vi "Sine_Trajectory_phase.vi"(6 "Phase(degrees)":dbl format="%0.2f", 7 "Amplitude":dbl, 8 "Offset":dbl, 9 "Frequency (Hz)":dbl, 10 "Duration (s)":dbl, 11 "Period (s)":dbl) -> (3 "Profile":cluster{"time (s)":dbl, "setpoint":dbl}[](array[cluster]) {"setpoint" format="%.2f"; "time (s)" format="%.3f"})   [LabVIEW 2015]
uses:
  <vilib>/Analysis/NI_AALBase.lvlib
panel:
  out "XY Graph":cluster{dbl, dbl}[](graph)
  # "Here needs to be 0.001 or so"
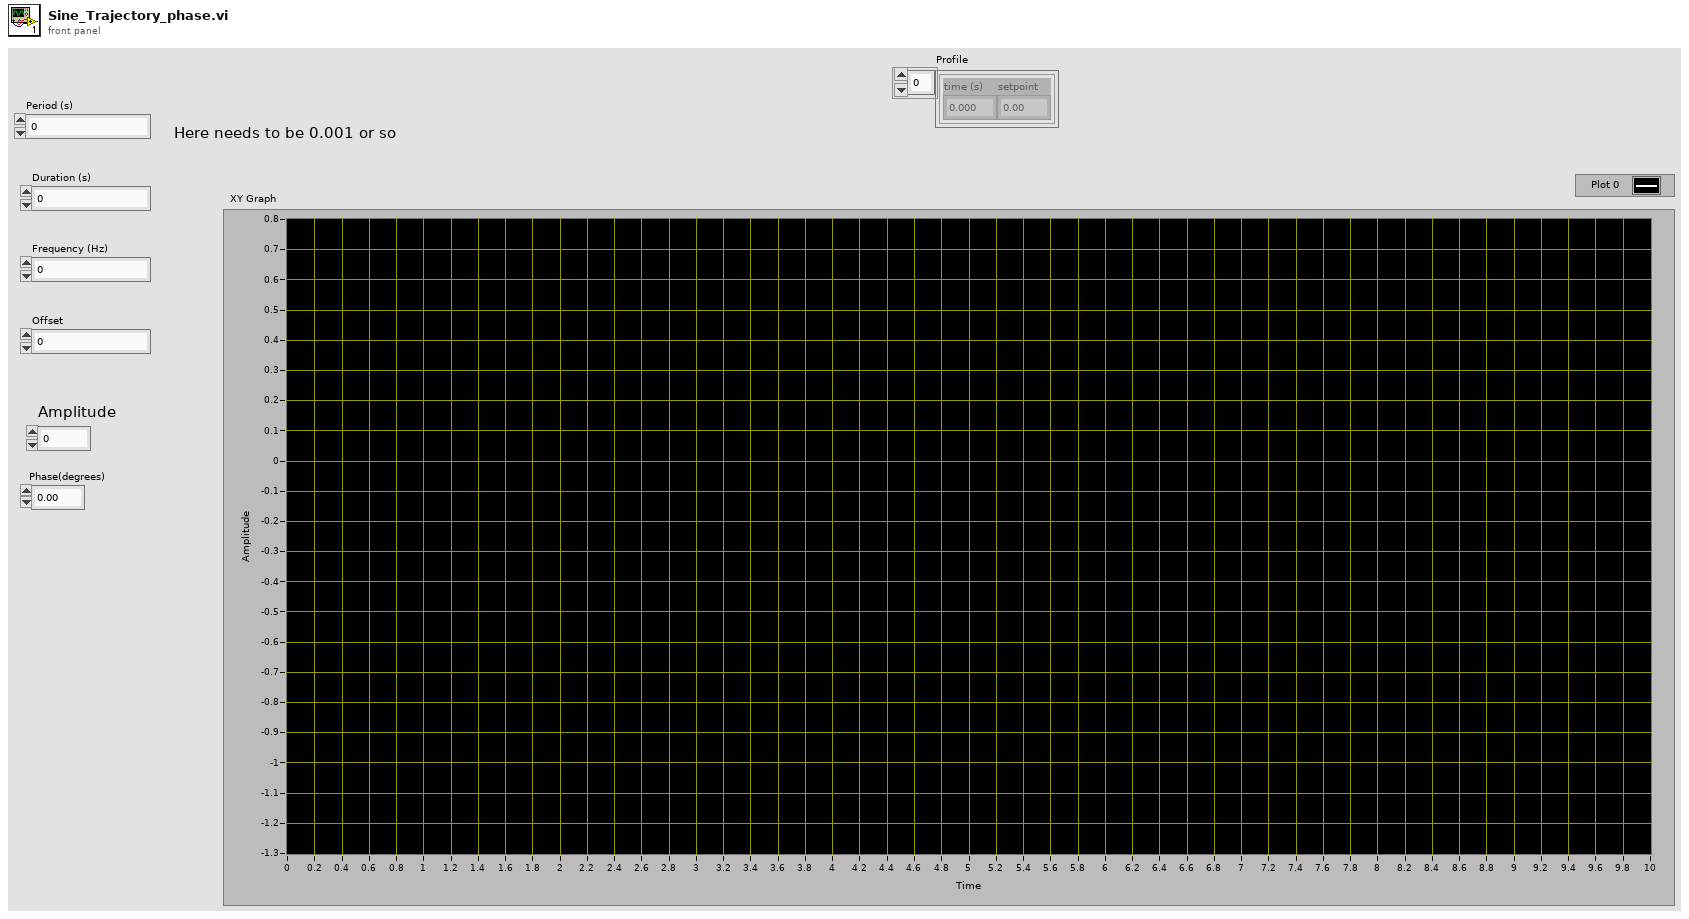
[diagram p1: front panel]
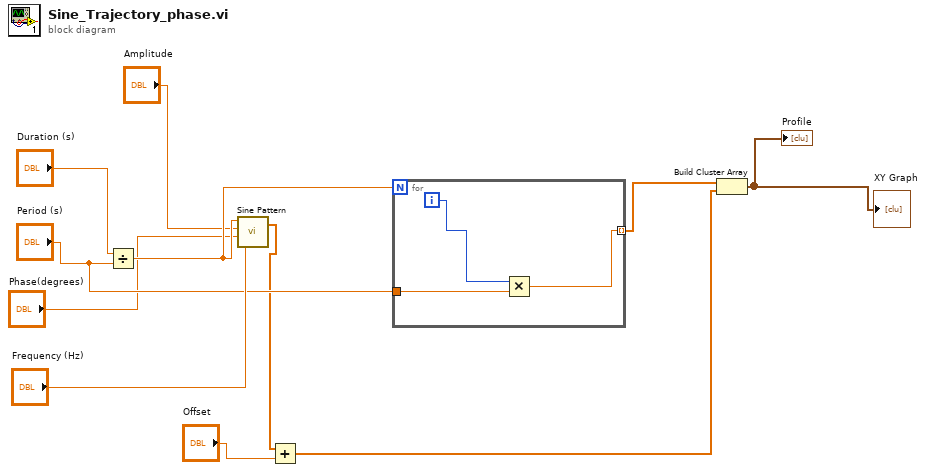
[diagram p0: block diagram]
diagram:
  n1 = Divide(x="Duration (s)", y="Period (s)") -> (x/y=w9:dbl)
  n2 = call <vilib>:"Sine Pattern.vi"("cycles"="Frequency (Hz)", "phase(degrees)"="Phase(degrees)", "amplitude"="Amplitude", "samples"=w9) -> ("Sinusoidal Pattern"=w4:dbl[])  [unwired: 1 out]
  n3 = Add(x=w4, y="Offset") -> (x+y=w3:dbl[])
  n4 = for {
    N: w9 -> [_]
    tunnel: [w12] -> w8 mode=indexing
    tunnel: "Period (s)" -> [w14]
    i -> [w13]
    n5 = Multiply(x=w13, y=w14) -> (x*y=w12:dbl)
  }
  n6 = Build Cluster Array(w8, w3) -> (→"XY Graph" →"Profile":cluster{dbl, dbl}[])
